vi "Set foyer.vi"(3 "cmd foyer sonde":bool caption="Ajuster le foyer de la \nsonde en conséquence ?", 4 "Foyer In":dbl format="%.2f") -> (0 "Foyer Out":dbl format="%.2f", 1 "DONE":bool, 2 "sortie foyer sonde":bool)   [LabVIEW 2019]
panel:
  in  "Bouton Annuler":bool
  in  "OK":bool
  in  "Foyer":dbl min=0.0 max=6000.0 step=1.0
  # "Assurrez-vous d'appuyer sur \"ENTER\" \n      pour confirmer la valeur entrée"
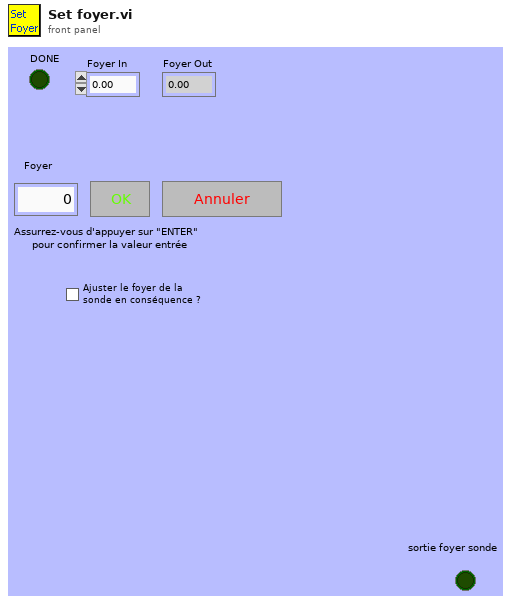
[diagram p1: front panel]
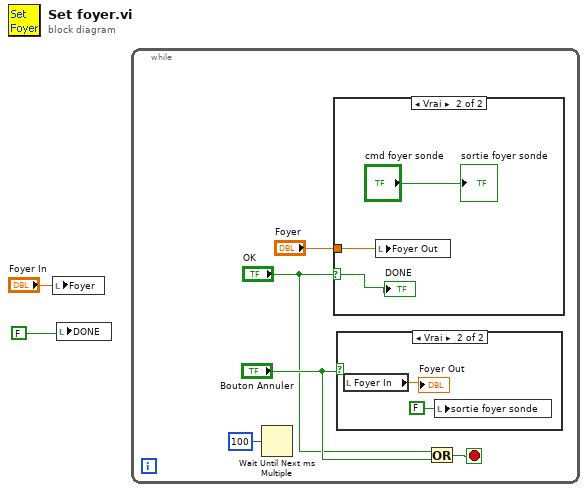
[diagram p0: block diagram]
diagram:
  n1 = local write "Foyer"("Foyer In") -> ()
  n2 = local write "DONE"(FALSE) -> ()
  n3 = while {
    stop <- w3 stop-if-true
    n4 = Wait Until Next ms Multiple(millisecond multiple=u32 100 ("n millisecondes")) -> ()  [unwired: 1 out]
    n5 = case shown="Vrai" "OK" {
      selector: "OK" -> [_ w11]
      tunnel: "Foyer" -> [_ w12]
      frame False {
      }
      frame True {
        n6 = local write "Foyer Out"(w12) -> ()
        "DONE" <- w11
        "sortie foyer sonde" <- "cmd foyer sonde"
      }
    }
    n7 = case shown="Vrai" "Bouton Annuler" {
      frame False {
      }
      frame True {
        n8 = local read "Foyer In"() -> (→"Foyer Out":dbl)
        n9 = local write "sortie foyer sonde"(FALSE ("sortie foyer sonde")) -> ()
      }
    }
    n10 = Or(x="OK", y="Bouton Annuler") -> (x .or. y?=w3:bool)
  }
